vi "TEST - Get Array Element Default Data.vi"(8 "error in (no error)":errorcluster) -> (0 "error out":errorcluster, 2 "pass":bool)   [LabVIEW 2013]
panel:
  out "Failures":T1(array[cluster])
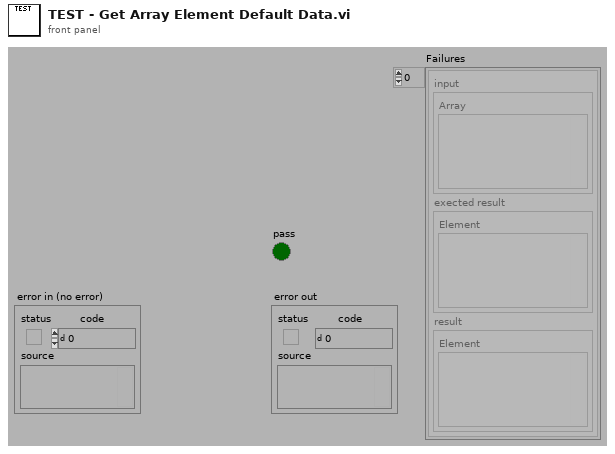
[diagram p1: front panel]
types:
  T1 = cluster{"input":cluster{"Array":variant}, "exected result":cluster{"Element":variant}, "result":cluster{"Element":variant}}[]
  T2 = cluster{"input":cluster{"Array":variant}, "exected result":cluster{"Element":variant}, "result":cluster{"Element":variant}}
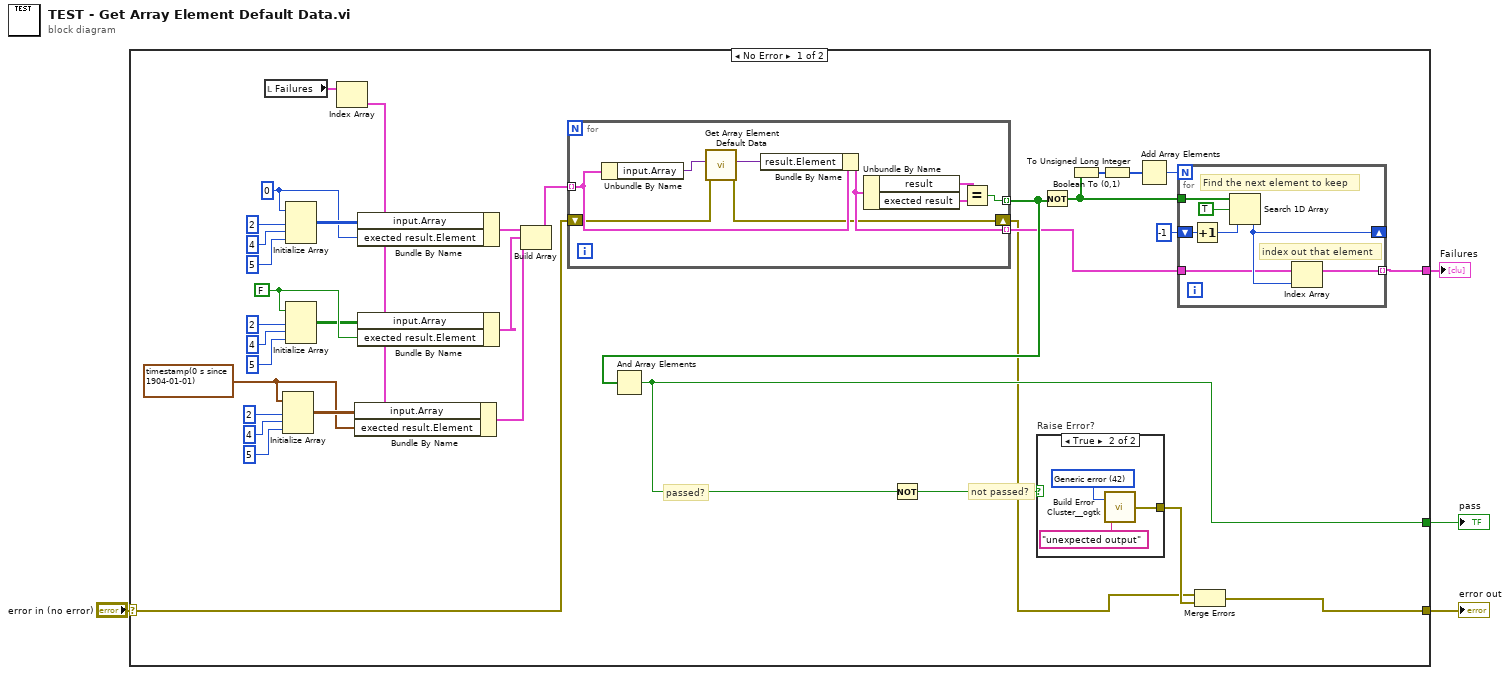
[diagram p0: block diagram]
diagram:
  n1 = case shown="No Error" "error in (no error)" {
    selector: "error in (no error)" -> [w25 w59]
    tunnel: [w36 _] -> w4
    tunnel: [w39 w59] -> w2
    tunnel: [w28 _] -> w1
    frame No Error {
      w7 = timestamp(0 s since 1904-01-01) ("Time Stamp")
      w17 = FALSE
      w18 = 0
      # "not passed?"
      # "passed?"
      n2 = local read "Failures"() -> (w23:T1)
      n3 = Initialize Array(w7, u32 2 ("Numeric"), 4 ("Numeric"), 5 ("Numeric")) -> (w8:timestamp[][][])
      n4 = Initialize Array(w18, u32 2 ("Numeric"), 4 ("Numeric"), 5 ("Numeric")) -> (w19:i32[][][])
      n5 = Initialize Array(w17, u32 2 ("Numeric"), 4 ("Numeric"), 5 ("Numeric")) -> (w16:bool[][][])
      n6 = Index Array(array=w23) -> (element=w5:T2)  [unwired: 1 in]
      n7 = Bundle By Name(cluster=w5, "input.Array"=w8, "exected result.Element"=w7) -> (w6:T2)
      n8 = Bundle By Name(cluster=w5, "input.Array"=w19, "exected result.Element"=w18) -> (w27:T2)
      n9 = Bundle By Name(cluster=w5, "input.Array"=w16, "exected result.Element"=w17) -> (w12:T2)
      n10 = Build Array(w27, w12, w6) -> (w26:T1)
      n11 = for {
        tunnel: w26 -> [w54] mode=indexing
        tunnel: [w55] -> w30 mode=indexing
        tunnel: [w53] -> w29 mode=indexing
        shift-right: [w49] -> w24
        shift-left: w25 -> [w50]
        n12 = Unbundle By Name(w54) -> ("input.Array"=w48:variant)
        n13 = call "Get Array Element Default Data.vi"("error in (no error)"=w50, "Array"=w48) -> ("error out"=w49:errorcluster, "Array Element Default Data"=w47:variant)  [unwired: 8 in]
        n14 = Bundle By Name(cluster=w54, "result.Element"=w47) -> (w53:T2)
        n15 = Unbundle By Name(w53) -> ("result"=w52:cluster{"Element":variant}, "exected result"=w51:cluster{"Element":variant})
        n16 = Equal?(x=w52, y=w51) -> (x = y?=w55:bool)
      }
      n17 = And Array Elements(Boolean array=w30) -> (logical AND=w36:bool)
      n18 = Not(x=w36) -> (.not. x?=w37:bool)
      n19 = case "Raise Error?" shown="True" w37 {
        tunnel: [_ w56] -> w38
        frame False {
        }
        frame True {
          w57 = 42 items=["No error", "Argument error", "Memory is full", "Out of zone", "End of file", "File already open", "Generic file I/O error", "File not found", "File permission error", "Disk is full", "Duplicate path", "Too many files open", "System feature not enabled", "Resource file not found", "Cannot add resource", "Resource not found", "Image not found", "Image memory error", "Pen does not exist", "Config type invalid", "Config token not found", "Config parse error", "Config memory error", "Bad external code format", "Bad external code offset", "External code not present", "Null window", "Destroy window error", "Null menu", "Print aborted", "Bad print record", "Print driver error", "Windows error during printing", "Memory error during printing", "Print dialog error", "Generic print error", "Invalid device refnum", "Device not found", "Device parameter error", "Device unit error", "Cannot open device", "Device call aborted", "Generic error", "Cancelled by user", "Object ID too low", "Object ID too high", "Object not in heap", "Unknown heap", "Unknown object (invalid DefProc)", "Unknown object (DefProc not in table)", "Message out of range", "Invalid (null) method", "Unknown message", "Manager call not supported", "Bad address", "Network operation in progress", "Network operation timed out", "Connection is busy", "Network attribute not supported", "Network error", "Address in use", "System out of memory", "Connection aborted", "Connection refused", "Not connected", "Already connected", "Connection closed", "Initialization error (interapplication manager)", "Bad occurrence", "Wait on unbound occurrence handler", "Occurrence queue overflow", "Datalog type conflict", "Unused", "Unrecognized type (interapplication manager)", "Memory corrupt", "Failed to make temporary DLL", "Old CIN version", "Drag socket not found", "Failed to load drop-object", "Failed to register OLE object", "Failed to release OLE object", "Format specifier type mismatch", "Unknown format specifier", "Too few format specifiers", "Too many format specifiers", "Scan failed", "Newer CIN version", "Error converting to variant", "Runtime menu error", "Password tampered", "Variant attribute not found", "Incompatible variant data type", "Event data is not available", "Event Store is not present", "Occurrence is not found", "Event Queue is not created", "Event info is not available", "Refnum passed is NULL", "Error retrieving Class GUID", "Error retrieving CoClass GUID", "Error retrieving TypeLib GUID.", "Bad built application magic bytes.", "Specific driver is different from the specific driver associated with the Logical Name.", "There is no session opened to the class driver.", "Max Error", "MAX - Error with config objects", "MAX - Error loading configuration", "MAX - Group not supported"]
          n20 = call <userlib>:"Build Error Cluster__ogtk.vi"("String to Prepend to source (\"\")"="unexpected output" ("String to Prepend to source (\"\")"), "code"=w57) -> ("error out"=w56:errorcluster)
        }
      }
      n21 = Not(x=w30) -> (.not. x?=w32:bool[])
      n22 = Boolean To (0,1)(Boolean=w32) -> (0, 1=w33:i16[])
      n23 = To Unsigned Long Integer(number=w33) -> (unsigned 32bit integer=w31:u32[])
      n24 = Add Array Elements(numeric array=w31) -> (sum=w34:u32)
      n25 = for {
        N: w34 -> [_]
        tunnel: w29 -> [w42]
        tunnel: w32 -> [w46]
        shift-right: [w43] -> _
        shift-left: -1 ("start index (0)") -> [w44]
        tunnel: [w41] -> w28 mode=indexing
        # "index out that element"
        # "Find the next element to keep"
        n26 = Increment(x=w44) -> (x+1=w40:i32)
        n27 = Search 1D Array(1D array=w46, element=TRUE, start index (0)=w40) -> (index of element=w43:i32)
        n28 = Index Array(array=w42, index=w43) -> (element=w41:T2)
      }
      n29 = Merge Errors(w24, w38) -> (w39:errorcluster)
    }
    frame Error {
    }
  }
  "pass" <- w4
  "error out" <- w2
  "Failures" <- w1
